vi "Terminal Type Matches RegExp.vi"   [LabVIEW 2012, in "Scripting Tools.lvlib" / "XNode Support.lvlib"]
uses:
  XNode Support.lvlib
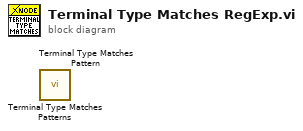
[diagram p0: block diagram]
diagram:
  n1 = call "Terminal Type Matches Patterns.vi"() -> ()  [unwired: 9 in, 3 out]
  n2 = call "Terminal Type Matches Pattern.vi"() -> ()  [unwired: 10 in, 2 out]
